vi "VI Tree - comparison__ogtk.vi"   [LabVIEW 2018]
uses:
  <userlib>/_OpenG.lib/comparison/comparison.llb/Variant Changed__ogtk.vi
panel:
  # "[OpenG VI Tags] ***Do Not Remove***"
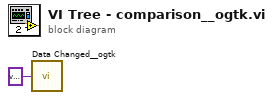
[diagram p0: block diagram]
diagram:
  n1 = call-poly <userlib>:"Data Changed__ogtk.vi"("Variant"=variant) -> ()  [unwired: 1 out]
